vi "Solve_Problem_with_Loosing_Elongations-1.vi"(3 "[IN] Indicies of Cross\nconnected Points":i32[](array[numeric]), 5 "[IN] Track group":T1) -> (2 "[OUT] Track group":T1)   [LabVIEW 2013]
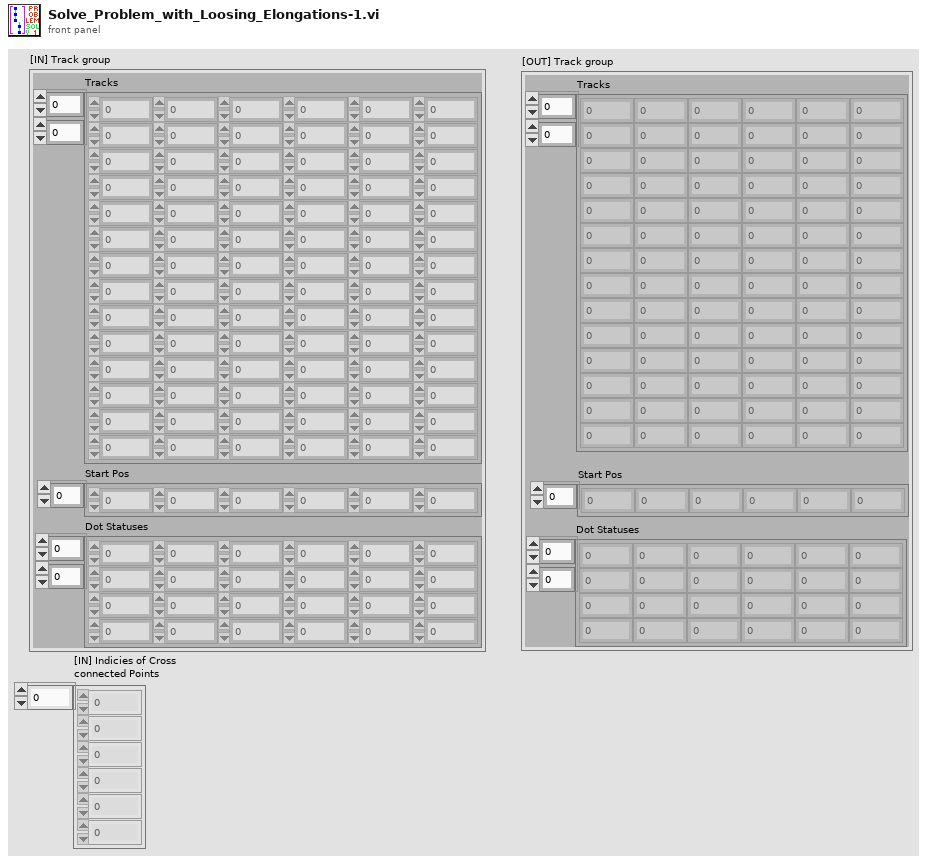
[diagram p1: front panel]
types:
  T1 = cluster{"Tracks":dbl[][], "Start Pos":i32[], "Dot Statuses":i16[][]}
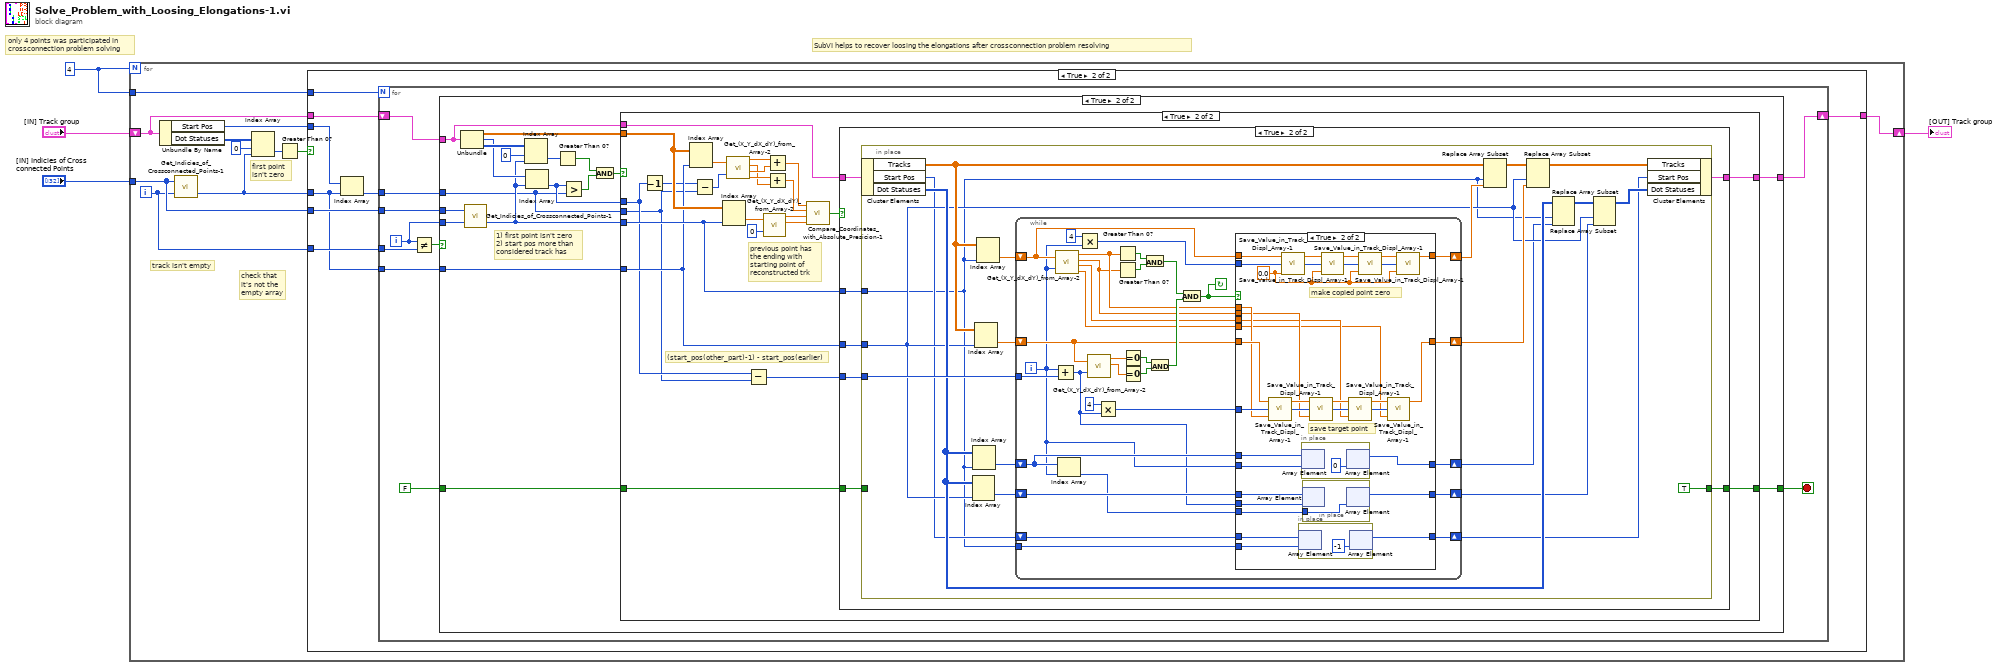
[diagram p0: block diagram]
diagram:
  w2 = 4
  # "only 4 points was participated in \ncrossconnection problem solving"
  # "SubVI helps to recover loosing the elongations after crossconnection problem resolving"
  n1 = for {
    N: w2 -> [_]
    tunnel: "[IN] Indicies of Cross\nconnected Points" -> [w8]
    tunnel: w2 -> [w9]
    shift-right: [w5] -> w1
    shift-left: "[IN] Track group" -> [w6]
    i -> [w7]
    # "track isn't empty"
    # "check that \nit's not the \nempty array"
    # "first point\nisn't zero"
    n2 = Unbundle By Name(w6) -> ("Start Pos"=w11:i32[], "Dot Statuses"=w15:i16[][])
    n3 = call "Get_Indicies_of_Crossconnected_Points-1.vi"("[IN] Index of point"=w7, "[IN] Indicies of Cross\nconnected Points"=w8) -> ("[OUT] Column index"=w10:i32)  [unwired: 1 out]
    n4 = Index Array(array=w15, index (row)=0 ("disabled index (row)"), index (col)=w10) -> (element=w13:i16)
    n5 = Greater Than 0?(x=w13) -> (x > 0?=w12:bool)
    n6 = case shown="True" w12 {
      tunnel: w11 -> [_ w20]
      tunnel: w10 -> [_ w18]
      tunnel: w9 -> [_ w24]
      tunnel: w8 -> [_ w22]
      tunnel: w7 -> [_ w21]
      tunnel: w6 -> [w16 w19]
      tunnel: [w16 w17] -> w5
      frame False {
      }
      frame True {
        n7 = Index Array(array=w20, index=w18) -> (element=w23:i32)
        n8 = for {
          N: w24 -> [_]
          tunnel: w23 -> [w30]
          tunnel: w22 -> [w32]
          tunnel: w21 -> [w34]
          shift-right: [w25] -> w17
          shift-left: w19 -> [w29]
          tunnel: w18 -> [w28]
          i -> [w31]
          stop <- w26 stop-if-true
          n9 = Not Equal?(x=w31, y=w34) -> (x != y?=w33:bool)
          n10 = case shown="True" w33 {
            tunnel: w32 -> [_ w54]
            tunnel: w31 -> [_ w53]
            tunnel: w30 -> [_ w37]
            tunnel: w29 -> [w35 w41]
            tunnel: w28 -> [_ w43]
            tunnel: FALSE -> [w36 w40]
            tunnel: [w36 w39] -> w26
            tunnel: [w35 w38] -> w25
            frame False {
            }
            frame True {
              # "1) first point isn't zero\n2) start pos more than \nconsidered track has"
              n11 = Unbundle(w41) -> ("Tracks"=w45:dbl[][], "Start Pos"=w49:i32[], "Dot Statuses"=w52:i16[][])
              n12 = call "Get_Indicies_of_Crossconnected_Points-1.vi"("[IN] Index of point"=w53, "[IN] Indicies of Cross\nconnected Points"=w54) -> ("[OUT] Column index"=w42:i32)  [unwired: 1 out]
              n13 = Index Array(array=w52, index (row)=0 ("disabled index (row)"), index (col)=w42) -> (element=w50:i16)
              n14 = Index Array(array=w49, index=w42) -> (element=w44:i32)
              n15 = Greater Than 0?(x=w50) -> (x > 0?=w48:bool)
              n16 = Greater?(x=w44, y=w37) -> (0:w47:bool)
              n17 = And(x=w48, y=w47) -> (x .and. y?=w46:bool)
              n18 = case shown="True" w46 {
                tunnel: w45 -> [_ w76]
                tunnel: w44 -> [_ w59]
                tunnel: w43 -> [_ w66]
                tunnel: w42 -> [_ w67]
                tunnel: w41 -> [w55 w68]
                tunnel: w40 -> [w56 w64]
                tunnel: [w56 w63] -> w39
                tunnel: [w55 w62] -> w38
                tunnel: w37 -> [_ w58]
                frame False {
                }
                frame True {
                  # "(start_pos(other_part)-1) - start_pos(earlier)"
                  # "previous point has\nthe ending with \nstarting point of \nreconstructed trk"
                  n19 = Decrement(x=w59) -> (x-1=w61:i32)
                  n20 = Index Array(array=w76, index (col)=w66) -> (element=w65:dbl[])  [unwired: 1 in]
                  n21 = Subtract(x=w61, y=w58) -> (x-y=w60:i32)
                  n22 = Index Array(array=w76, index (col)=w67) -> (element=w75:dbl[])  [unwired: 1 in]
                  n23 = call "Get_(X_Y_dX_dY)_from_Array-2.vi"("(X,Y,dX,dY)"=w65, "Index of Displacement"=w60) -> ("X"=w80:dbl, "Y"=w77:dbl, "dX"=w79:dbl, "dY"=w78:dbl)
                  n24 = Subtract(x=w59, y=w58) -> (x-y=w57:i32)
                  n25 = call "Get_(X_Y_dX_dY)_from_Array-2.vi"("(X,Y,dX,dY)"=w75, "Index of Displacement"=0) -> ("X"=w73:dbl, "Y"=w72:dbl)  [unwired: 2 out]
                  n26 = Add(x=w80, y=w79) -> (x+y=w71:dbl)
                  n27 = Add(x=w78, y=w77) -> (x+y=w70:dbl)
                  n28 = call "Compare_Coordinates_with_Absolute_Presicion-1.vi"("X 1"=w71, "Y 1"=w70, "X 2"=w73, "Y 2"=w72) -> ("[OUT] Same coordinates?"=w69:bool)  [unwired: 1 in]
                  n29 = case shown="True" w69 {
                    tunnel: w68 -> [w81 w89]
                    tunnel: w67 -> [_ w88]
                    tunnel: w66 -> [_ w87]
                    tunnel: w57 -> [_ w86]
                    tunnel: w64 -> [w82 w85]
                    tunnel: [w81 w84] -> w62
                    tunnel: [w82 w83] -> w63
                    frame False {
                    }
                    frame True {
                      n30 = in-place {
                        in-place-border: w88 -> [w91]
                        in-place-border: w87 -> [w96]
                        in-place-border: w86 -> [w107]
                        in-place-border: w85 -> [_]
                        in-place-border: [TRUE] -> w83
                        n31 = in-place-cluster #1(w89) -> ("Tracks"=w104:dbl[][], "Start Pos"=w92:i32[], "Dot Statuses"=w99:i16[][])
                        n32 = Index Array(array=w99, index (col)=w96) -> (element=w105:i16[])  [unwired: 1 in]
                        n33 = Index Array(array=w99, index (col)=w91) -> (element=w106:i16[])  [unwired: 1 in]
                        n34 = Index Array(array=w104, index (col)=w96) -> (element=w109:dbl[])  [unwired: 1 in]
                        n35 = Index Array(array=w104, index (col)=w91) -> (element=w108:dbl[])  [unwired: 1 in]
                        n36 = while {
                          shift-right: [w120] -> w101
                          shift-left: w109 -> [w126]
                          shift-right: [w121] -> w103
                          shift-left: w108 -> [w129]
                          tunnel: w107 -> [w140]
                          shift-right: [w118] -> w93
                          shift-left: w106 -> [w119]
                          shift-right: [w114] -> w97
                          shift-left: w105 -> [w117]
                          shift-right: [w110] -> w90
                          shift-left: w92 -> [w112]
                          tunnel: w91 -> [w111]
                          i -> [w116]
                          stop <- w130 continue-if-true
                          n37 = Add(x=w116, y=w140) -> (x+y=w113:i32)
                          n38 = call "Get_(X_Y_dX_dY)_from_Array-2.vi"("(X,Y,dX,dY)"=w129, "Index of Displacement"=w116) -> ("X"=w125:dbl, "Y"=w124:dbl, "dX"=w123:dbl, "dY"=w122:dbl)
                          n39 = Index Array(array=w119, index=w116) -> (element=w115:i16)
                          n40 = Multiply(x=4, y=w116) -> (x*y=w128:i32)
                          n41 = call "Get_(X_Y_dX_dY)_from_Array-2.vi"("(X,Y,dX,dY)"=w126, "Index of Displacement"=w113) -> ("X"=w139:dbl, "Y"=w138:dbl)  [unwired: 2 out]
                          n42 = Multiply(x=4, y=w113) -> (x*y=w127:i32)
                          n43 = Greater Than 0?(x=w125) -> (x > 0?=w135:bool)
                          n44 = Greater Than 0?(x=w124) -> (x > 0?=w134:bool)
                          n45 = Equal To 0?(x=w139) -> (x = 0?=w137:bool)
                          n46 = Equal To 0?(x=w138) -> (x = 0?=w136:bool)
                          n47 = And(x=w135, y=w134) -> (x .and. y?=w132:bool)
                          n48 = And(x=w137, y=w136) -> (x .and. y?=w133:bool)
                          n49 = And(x=w132, y=w133) -> (x .and. y?=w130:bool)
                          n50 = case shown="True" w130 {
                            tunnel: w129 -> [w146 w179]
                            tunnel: w128 -> [_ w178]
                            tunnel: w127 -> [_ w170]
                            tunnel: w126 -> [w145 w169]
                            tunnel: w125 -> [_ w168]
                            tunnel: w124 -> [_ w165]
                            tunnel: w123 -> [_ w162]
                            tunnel: w122 -> [_ w159]
                            tunnel: [w146 w158] -> w121
                            tunnel: [w145 w157] -> w120
                            tunnel: w119 -> [w144 w156]
                            tunnel: [w144 w155] -> w118
                            tunnel: w116 -> [_ w154]
                            tunnel: w117 -> [w143 w153]
                            tunnel: w113 -> [_ w152]
                            tunnel: w115 -> [_ w151]
                            tunnel: [w143 w150] -> w114
                            tunnel: w112 -> [w142 w149]
                            tunnel: w111 -> [_ w148]
                            tunnel: [w142 w147] -> w110
                            frame False {
                            }
                            frame True {
                              w171 = 0.0 ("[IN] Value")
                              # "save target point"
                              # "make copied point zero"
                              n51 = call "Save_Value_in_Track_Displ_Array-1.vi"("[IN] Value"=w168, "[IN] Index"=w170, "[IN] Empty tracks\nfor points saving"=w169) -> ("[OUT] Index ++"=w166:i32, "[OUT Track with saved value"=w167:dbl[])  [unwired: 1 in]
                              n52 = call "Save_Value_in_Track_Displ_Array-1.vi"("[IN] Value"=w171, "[IN] Index"=w178, "[IN] Empty tracks\nfor points saving"=w179) -> ("[OUT] Index ++"=w176:i32, "[OUT Track with saved value"=w177:dbl[])  [unwired: 1 in]
                              n53 = in-place {
                                n54 = in-place-array #2(w149, w148) -> ()  [unwired: 1 out]
                                n55 = in-place-array #2(-1) -> (w147:i32[])  [unwired: 1 out]
                              }
                              n56 = in-place {
                                n57 = in-place-array #3(w156, w154) -> ()  [unwired: 1 out]
                                n58 = in-place-array #3(i16 0) -> (w155:i16[])  [unwired: 1 out]
                              }
                              n59 = in-place {
                                in-place-border: w151 -> [w181]
                                n60 = in-place-array #4(w153, w152) -> ()  [unwired: 1 out]
                                n61 = in-place-array #4(w181) -> (w150:i16[])  [unwired: 1 out]
                              }
                              n62 = call "Save_Value_in_Track_Displ_Array-1.vi"("[IN] Value"=w165, "[IN] Index"=w166, "[IN] Empty tracks\nfor points saving"=w167) -> ("[OUT] Index ++"=w163:i32, "[OUT Track with saved value"=w164:dbl[])  [unwired: 1 in]
                              n63 = call "Save_Value_in_Track_Displ_Array-1.vi"("[IN] Value"=w171, "[IN] Index"=w176, "[IN] Empty tracks\nfor points saving"=w177) -> ("[OUT] Index ++"=w174:i32, "[OUT Track with saved value"=w175:dbl[])  [unwired: 1 in]
                              n64 = call "Save_Value_in_Track_Displ_Array-1.vi"("[IN] Value"=w162, "[IN] Index"=w163, "[IN] Empty tracks\nfor points saving"=w164) -> ("[OUT] Index ++"=w160:i32, "[OUT Track with saved value"=w161:dbl[])  [unwired: 1 in]
                              n65 = call "Save_Value_in_Track_Displ_Array-1.vi"("[IN] Value"=w171, "[IN] Index"=w174, "[IN] Empty tracks\nfor points saving"=w175) -> ("[OUT] Index ++"=w172:i32, "[OUT Track with saved value"=w173:dbl[])  [unwired: 1 in]
                              n66 = call "Save_Value_in_Track_Displ_Array-1.vi"("[IN] Value"=w159, "[IN] Index"=w160, "[IN] Empty tracks\nfor points saving"=w161) -> ("[OUT Track with saved value"=w157:dbl[])  [unwired: 1 in, 1 out]
                              n67 = call "Save_Value_in_Track_Displ_Array-1.vi"("[IN] Value"=w171, "[IN] Index"=w172, "[IN] Empty tracks\nfor points saving"=w173) -> ("[OUT Track with saved value"=w158:dbl[])  [unwired: 1 in, 1 out]
                            }
                          }
                        }
                        n68 = Replace Array Subset(array=w104, new element=w103, index (col)=w91) -> (w102:dbl[][])  [unwired: 1 in]
                        n69 = Replace Array Subset(array=w102, new element=w101, index (col)=w96) -> (w100:dbl[][])  [unwired: 1 in]
                        n70 = Replace Array Subset(array=w99, new element=w93, index (col)=w91) -> (w98:i16[][])  [unwired: 1 in]
                        n71 = Replace Array Subset(array=w98, new element=w97, index (col)=w96) -> (w95:i16[][])  [unwired: 1 in]
                        n72 = in-place-cluster #1("Tracks"=w100, "Start Pos"=w90, "Dot Statuses"=w95) -> (w84:T1)
                      }
                    }
                  }
                }
              }
            }
          }
        }
      }
    }
  }
  "[OUT] Track group" <- w1
